vi "DeviceOff.vi"(8 "error in (no error)":errorcluster, 11 "NHRDCPower in":refnum<class "NHRDCPower.lvclass">) -> (0 "error out":errorcluster, 3 "NHRDCPower out":refnum<class "NHRDCPower.lvclass">)   [LabVIEW 2018, in "AcPwrPlugins.lvlib" / "NHRDCPower.lvclass"]
doc: "This VI disables the instruments output form either generating or receiving a signal."
uses:
  NHRDCPower.lvclass
  <instrlib>/NHRDCPowerModule/NHRDCPowerModule/NHRDCPowerModule.lvlib
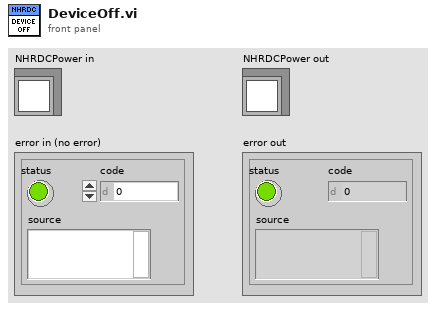
[diagram p1: front panel]
types:
  T1 = typedef "AcPwrPlugins.lvlib/NHRDCPower.lvclass/Modules.ctl" = cluster{"Handle":string, "Name":string, "id query (Yes)":bool, "reset device (Yes)":bool, "Connected":bool, "Initial Battery Detect Voltage (0)":dbl, "SafetySettings":cluster{"SetWatchDog?":bool, "Voltage (V)":dbl, "Current (A)":dbl, "Power (W)":dbl, "Voltage Delay (s)":dbl, "Current Delay (s)":dbl, "Power Delay (s)":dbl}, "Options String":string, "Aperture Time (s)":dbl, "operating state (Off)":i32, "OutputSettings":cluster{"Voltage (V)":dbl, "Current (A)":dbl, "Resistance (Ohms)":dbl, "Power (W)":dbl, "Enable Voltage":bool, "Enable Current":bool, "Enable Resistance":bool, "Enable Power":bool, "Macro After Step Delay  (s)":dbl, "Wait Value (V, A, W)":dbl, "Enable Wait":bool, "Wait on Value":i32}[], "SlewRate":cluster{"Set Voltage Rate V/S":dbl, "Set Current Rate A/S":dbl, "Set Resistance Rate R/S":dbl, "Set Power Rate W/S":dbl}, "Macro":cluster{"Save Macro?":bool, "Load Macro From File?":bool, "Run Macro Continuously?":bool, "Use Macros?":bool, "Load Macro File Path":string, "Save Macro File Path":string}, "Regulation Gain (1=100%)":dbl, "UpdatingOntheFly":bool}[]
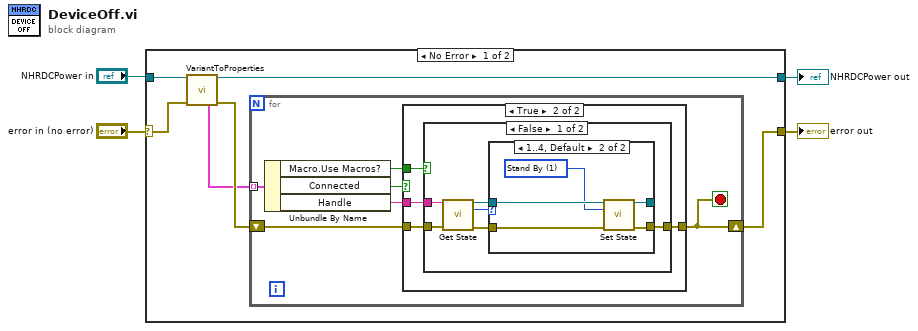
[diagram p0: block diagram]
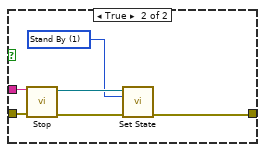
[diagram p4: hidden frame]
diagram:
  n1 = case shown="No Error" "error in (no error)" {
    selector: "error in (no error)" -> [w6 w42]
    tunnel: [w10 w42] -> w1
    tunnel: [w8 w41] -> w2
    tunnel: "NHRDCPower in" -> [w7 w41]
    frame No Error {
      n2 = call "VariantToProperties.vi"("NHRDCPower in"=w7, "error in (no error)"=w6) -> ("NHRDCPower out"=w8:refnum<class "NHRDCPower.lvclass">, "Modules"=w5:T1, "error out"=w9:errorcluster)  [unwired: 7 in, 4 out]
      n3 = for {
        tunnel: w5 -> [w16] mode=indexing
        shift-right: [w14] -> w10
        shift-left: w9 -> [w15]
        stop <- w14 stop-if-true
        n4 = Unbundle By Name(w16) -> ("Macro.Use Macros?"=w11:bool, "Connected"=w12:bool, "Handle"=w13:string)
        n5 = case shown="True" w12 {
          tunnel: w15 -> [w17 w19]
          tunnel: [w17 w21] -> w14
          tunnel: w13 -> [_ w20]
          tunnel: w11 -> [_ w18]
          frame False {
          }
          frame True {
            n6 = case shown="False" w18 {
              tunnel: [w27 w37] -> w21
              tunnel: w20 -> [w26 w39]
              tunnel: w19 -> [w25 w40]
              frame False {
                n7 = call <instrlib>:"Get State.vi"("instrument handle"=w26, "error in (no error)"=w25) -> ("instrument handle out"=w22:refnum<visa-resource-name>, "operating state"=w23:i32, "error out"=w24:errorcluster)  [unwired: 3 in, 8 out]
                n8 = case shown="1..4, Default" w23 {
                  tunnel: [w29 w33] -> w27
                  tunnel: w24 -> [w29 w34]
                  tunnel: w22 -> [w28 w32]
                  tunnel: [w28 w30] -> _
                  frame 0 {
                  }
                  frame 1..4, Default {
                    w31 = 1 items=["Off", "Stand By", "Charge", "Discharge", "Battery Emulation"] ("operating state (Off)")
                    n9 = call <instrlib>:"Set State.vi"("instrument handle"=w32, "operating state (Off)"=w31, "error in (no error)"=w34) -> ("instrument handle out"=w30:refnum<visa-resource-name>, "error out"=w33:errorcluster)  [unwired: 11 in]
                  }
                }
              }
              frame True {
                w35 = 1 items=["Off", "Stand By", "Charge", "Discharge", "Battery Emulation"] ("operating state (Off)")
                n10 = call <instrlib>:"Stop.vi"("error in (no error)"=w40, "instrument handle"=w39) -> ("error out"=w38:errorcluster, "instrument handle out"=w36:refnum<visa-resource-name>)  [unwired: 8 in]
                n11 = call <instrlib>:"Set State.vi"("instrument handle"=w36, "operating state (Off)"=w35, "error in (no error)"=w38) -> ("error out"=w37:errorcluster)  [unwired: 11 in, 1 out]
              }
            }
          }
        }
      }
    }
    frame Error {
    }
  }
  "error out" <- w1
  "NHRDCPower out" <- w2
